vi "SHA-1 Digest.vi"(0 "s1":u32 format="%.0x", 5 "s2":u32 format="%.0x", 7 "s3":u32 format="%.0x", 9 "s4":u32 format="%.0x", 11 "s5":u32 format="%.0x") -> (4 "message-digest":u8[](array[numeric]))   [LabVIEW 2014, in "QwaveSys RPi Training Library.lvlib" / "WebSockets.lvlib"]
doc: "This VI performs certain bitwise operations on the state variables and converts them to hex strings such that they can be concatenated and displayed as the MD5 message-digest.\nWebSockets API 1.3.0.13\nSam Sharp - Intelligent Energy\nCopyright (c) 2015, Intelligent Energy"
uses:
  <vilib>/Q-Wave Systems/QwaveSys RPi Training Package (Demo)/Addons/WebSockets API/WebSockets/WebSockets.lvlib
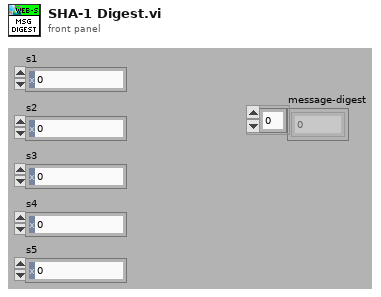
[diagram p1: front panel]
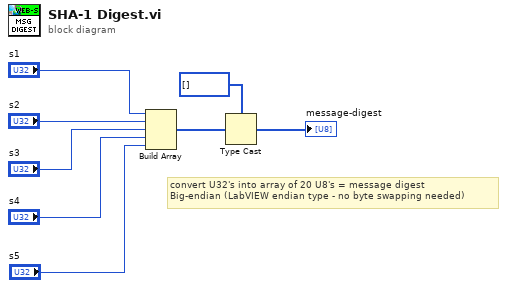
[diagram p0: block diagram]
diagram:
  # "convert U32's into array of 20 U8's = message digest\nBig-endian (LabVIEW endian type - no byte swapping needed)"
  n1 = Build Array("s1", "s2", "s3", "s4", "s5") -> (w3:u32[])
  n2 = Type Cast(type=u8[] [] ("message-digest 2"), x=w3) -> (*(type *) &x=→"message-digest":u8[])
